vi "GetName.vi"(8 "error in (no error)":errorcluster, 11 "text item in":refnum<class "text item.lvclass">) -> (0 "error out":errorcluster, 2 "name":string, 3 "text item out":refnum<class "text item.lvclass">)   [LabVIEW 2009, in "text item.lvclass"]
uses:
  text item.lvclass
  text item.lvclass/text item.ctl
  Text/text.lvclass
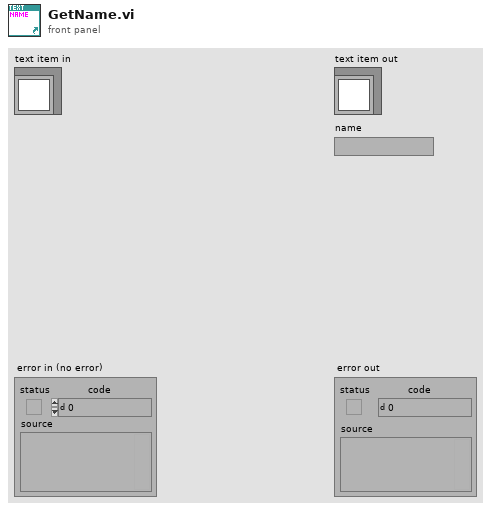
[diagram p1: front panel]
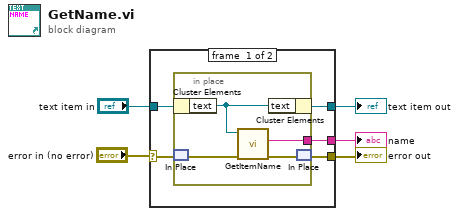
[diagram p0: block diagram]
diagram:
  n1 = case shown="No Error" "error in (no error)" {
    selector: "error in (no error)" -> [w6 w16]
    tunnel: [w7 w16] -> w4
    tunnel: "text item in" -> [w10 w15]
    tunnel: [w9 w15] -> w2
    tunnel: [w8 _] -> w1
    frame #0 {
      n2 = in-place {
        in-place-border: [w13] -> w8
        n3 = in-place-cluster #1(w10) -> ("text"=w14:refnum<class "text.lvclass">)
        n4 = in-place-match #2(w6) -> (w12:errorcluster)
        n5 = call "GetItemName.vi"("error in (no error)"=w12, "text in"=w14) -> ("error out"=w11:errorcluster, "item name"=w13:string)  [unwired: 7 in, 1 out]
        n6 = in-place-cluster #1("text"=w14) -> (w9:refnum<class "text item.lvclass">)
        n7 = in-place-match #2(w11) -> (w7:errorcluster)
      }
    }
    frame #1 {
    }
  }
  "text item out" <- w2
  "error out" <- w4
  "name" <- w1
